vi "EnableDisableSkipfire - Right Click.vi"(8 "error in (no error)":errorcluster, 11 "Node Ptr":u64 format="%.0x") -> (0 "error out":errorcluster)   [LabVIEW 2016, in "DCM System Explorer.lvlib"]
uses:
  DCM System Explorer.lvlib
  System.Windows.Forms
  Shared/DCM Constants and GUIDs.vi
  Shared/DCM Properties.vi
  <vilib>/NI Veristand/Custom Device API/Set Item Property (Boolean).vi
  <vilib>/NI VeriStand/Custom Device API/Custom Device API.lvlib
  DCM Shared.lvlib
  <vilib>/NI Veristand/Custom Device Tools/Custom Device Utility Library/Custom Device Utility Library.lvlib
panel:
  in  "Tag":string
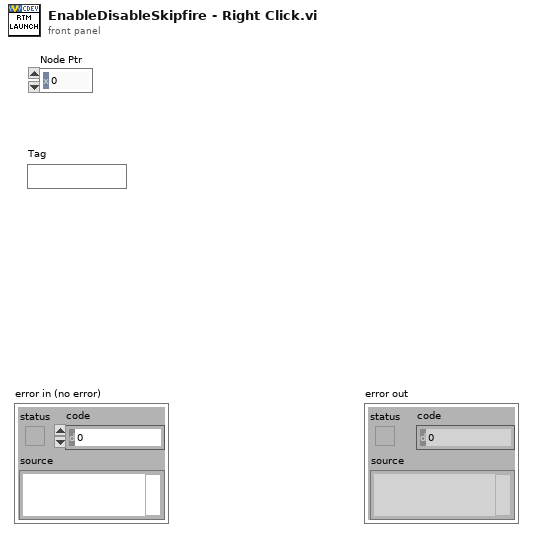
[diagram p1: front panel]
types:
  T1 = typedef "Custom Device API.lvlib/Custom Device Item Ref.ctl" = u64
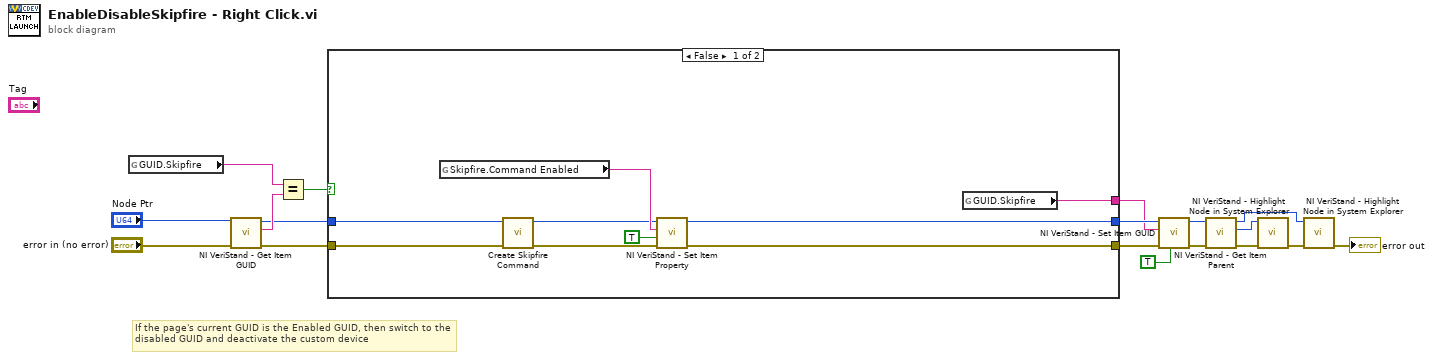
[diagram p0: block diagram]
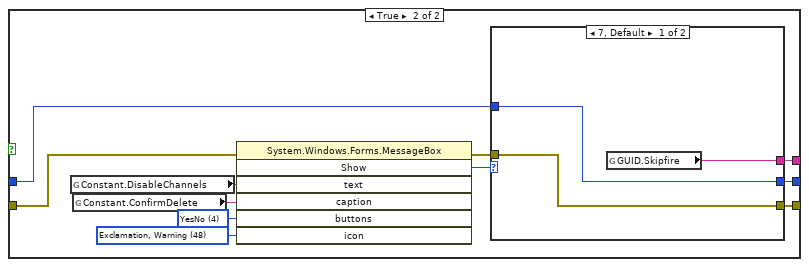
[diagram p2: hidden frame]
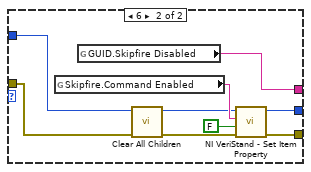
[diagram p3: hidden frame]
diagram:
  # "If the page's current GUID is the Enabled GUID, then switch to the disabled GUID and deactivate the custom device"
  n1 = global read "DCM Constants and GUIDs.vi" "GUID.Skipfire"() -> (w15:string)
  n2 = call <vilib>:"NI VeriStand - Get Item GUID.vi"("error in (no error)"="error in (no error)", "Item Ref in"="Node Ptr") -> ("error out"=w13:errorcluster, "GUID"=w18:string, "Item Ref out"=w14:T1)  [unwired: 7 in]
  n3 = Equal?(x=w15, y=w18) -> (x = y?=w1:bool)
  n4 = case shown="False" w1 {
    tunnel: w13 -> [w21 w34]
    tunnel: [w25 w31] -> w10
    tunnel: w14 -> [w22 w30]
    tunnel: [w24 w28] -> w11
    tunnel: [w23 w29] -> w9
    frame False {
      n5 = global read "DCM Properties.vi" "Skipfire.Command Enabled"() -> (w27:string)
      n6 = call "Create Skipfire Command.vi"("error in (no error)"=w21, "Section Ptr"=w22) -> ("error out"=w19:errorcluster, "Parent Ref out"=w20:T1)  [unwired: 8 in]
      n7 = call-poly <vilib>:"NI VeriStand - Set Item Property.vi"("error in (no error)"=w19, "Value"=TRUE, "Property Name"=w27, "Item Ref in"=w20) -> ("error out"=w25:errorcluster, "Item Ref out"=w24:T1)  [unwired: 5 in, 1 out]
      n8 = global read "DCM Constants and GUIDs.vi" "GUID.Skipfire"() -> (w23:string)
    }
    frame True {
      w35 = 4 items=["OK", "OKCancel", "AbortRetryIgnore", "YesNoCancel", "YesNo", "RetryCancel"] ("buttons")
      w36 = 48 items=["None"=0, "Hand, Error, Stop"=16, "Question"=32, "Exclamation, Warning"=48, "Asterisk, Information"=64] ("icon")
      n9 = global read "DCM Constants and GUIDs.vi" "Constant.DisableChannels"() -> (w37:string)
      n10 = global read "DCM Constants and GUIDs.vi" "Constant.ConfirmDelete"() -> (w38:string)
      n11 = invoke class="System.Windows.Forms.MessageBox" method="Show"(error in=w34, "text"=w37, "caption"=w38, "buttons"=w35, "icon"=w36) -> (error out=w32:errorcluster, "Show"=w33:i32)  [unwired: 2 in, 5 out]
      n12 = case shown="7, Default" w33 {
        tunnel: w32 -> [w41 w50]
        tunnel: [w41 w47] -> w31
        tunnel: w30 -> [w39 w49]
        tunnel: [w40 w43] -> w29
        tunnel: [w39 w42] -> w28
        frame 7, Default {
          n13 = global read "DCM Constants and GUIDs.vi" "GUID.Skipfire"() -> (w40:string)
        }
        frame 6 {
          n14 = global read "DCM Properties.vi" "Skipfire.Command Enabled"() -> (w46:string)
          n15 = global read "DCM Constants and GUIDs.vi" "GUID.Skipfire Disabled"() -> (w43:string)
          n16 = call "Clear All Children.vi"("error in (no error)"=w50, "Item Ref in"=w49) -> ("error out"=w48:errorcluster, "Item Ref out"=w44:T1)  [unwired: 8 in]
          n17 = call-poly <vilib>:"NI VeriStand - Set Item Property.vi"("error in (no error)"=w48, "Value"=FALSE, "Property Name"=w46, "Item Ref in"=w44) -> ("error out"=w47:errorcluster, "Item Ref out"=w42:T1)  [unwired: 5 in, 1 out]
        }
      }
    }
  }
  n18 = call <vilib>:"NI VeriStand - Set Item GUID.vi"("Refresh System Explorer Tree? (F)"=TRUE, "error in (no error)"=w10, "GUID"=w9, "Item Ref in"=w11) -> ("error out"=w6:errorcluster, "Item Ref out"=w5:T1)  [unwired: 6 in]
  n19 = call <vilib>:"NI VeriStand - Get Item Parent.vi"("error in (no error)"=w6, "Item Ref in"=w5) -> ("error out"=w7:errorcluster, "Parent Ref"=w8:T1, "Item Ref out"=w2:T1)  [unwired: 6 in, 1 out]
  n20 = call <vilib>:"NI VeriStand - Highlight Node in System Explorer.vi"("error in (no error)"=w7, "Item Ref in"=w8) -> ("error out"=w4:errorcluster)  [unwired: 8 in, 1 out]
  n21 = call <vilib>:"NI VeriStand - Highlight Node in System Explorer.vi"("error in (no error)"=w4, "Item Ref in"=w2) -> ("error out"=→"error out":errorcluster)  [unwired: 8 in, 1 out]
